vi "GPIO_RegChangeID.vi"(9 "GPIO Register New":T1, 11 "GPIO Register Old":T1) -> (1 "GPIO Reg Value":u32 format="%.0x", 3 "Command String":string)   [LabVIEW 2010]
doc: "This VI determines the GPIO data or direction bit that was change and creates the correct command string.\n\nInputs:\nGPIO Register Old - (cluster) previous value of GPIO register control\nGPIO Register New - (cluster) new value of GPIO register control\n\nOutputs:\nCommand String - (str) command for enqueue\n - for data bit change => \"GPIO Data Change:GPIODx\"\n - for direction bit change => \"GPIO Direction Change:GPIOCx\"\nGPIO Reg Value - (u32) GPIO regiter value"
uses:
  Controls/Register/TYP_Reg_GPIO.ctl
panel:
  out "GPIODx":u32
  out "GPIOCx":u32
  out "GPIODx Change?":bool caption="GPIODx Change? (or GPIOCx)"
  # "Out"
  # "IN"
  # "Out"
  # "IN"
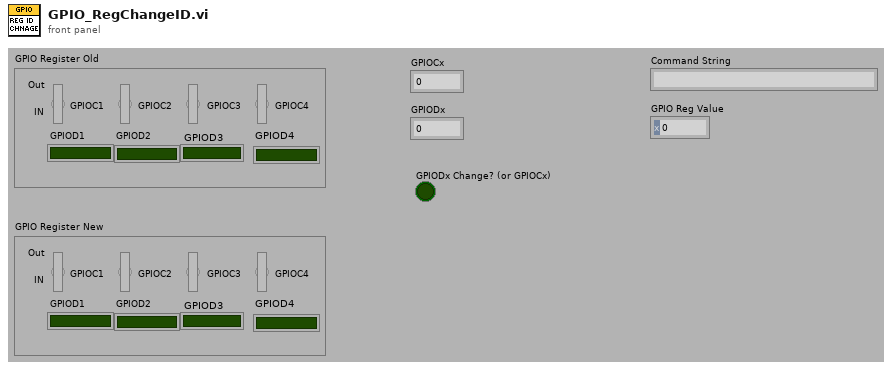
[diagram p1: front panel]
types:
  T1 = typedef "TYP_Reg_GPIO.ctl" = cluster{"GPIOC1":bool, "GPIOC2":bool, "GPIOC3":bool, "GPIOC4":bool, "GPIOD1":bool, "GPIOD2":bool, "GPIOD3":bool, "GPIOD4":bool}
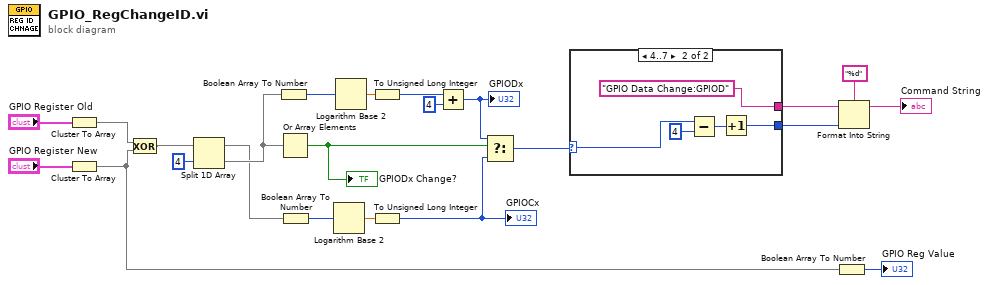
[diagram p0: block diagram]
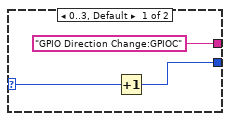
[diagram p2: hidden frame]
diagram:
  n1 = Cluster To Array(cluster="GPIO Register Old") -> (array=w14:bool[])
  n2 = Cluster To Array(cluster="GPIO Register New") -> (array=w2:bool[])
  n3 = Exclusive Or(1:w2, 2:w14) -> (0:w3:bool[])
  n4 = Split 1D Array(array=w3, index=4) -> (first subarray=w12:bool[], second subarray=w13:bool[])
  n5 = Boolean Array To Number(Boolean array=w13) -> (number=w20:u32)
  n6 = Or Array Elements(Boolean array=w13) -> (logical OR=w11:bool)
  "GPIODx Change?" <- w11
  n7 = Boolean Array To Number(Boolean array=w12) -> (number=w18:u32)
  n8 = Logarithm Base 2(1:w18) -> (0:w17:dbl)
  n9 = Logarithm Base 2(1:w20) -> (0:w19:dbl)
  n10 = To Unsigned Long Integer(number=w19) -> (unsigned 32bit integer=w16:u32)
  n11 = To Unsigned Long Integer(number=w17) -> (unsigned 32bit integer=w9:u32)
  "GPIOCx" <- w9
  n12 = Add(x=w16, y=u32 4) -> (x+y=w10:u32)
  "GPIODx" <- w10
  n13 = Select(t=w10, s=w11, f=w9) -> (s? t:f=w8:u32)
  n14 = case shown="4..7" w8 {
    selector: w8 -> [w26 w31]
    tunnel: [w25 w28] -> w7
    tunnel: ["GPIO Direction Change:GPIOC" "GPIO Data Change:GPIOD"] -> w6
    frame 0..3, Default {
      n15 = Increment(x=w26) -> (x+1=w25:u32)
    }
    frame 4..7 {
      n16 = Subtract(x=w31, y=u32 4) -> (x-y=w29:u32)
      n17 = Increment(x=w29) -> (x+1=w28:u32)
    }
  }
  n18 = Boolean Array To Number(Boolean array=w2) -> (number=→"GPIO Reg Value":u32)
  n19 = Format Into String(format string="%d", initial string=w6, w7) -> (resulting string=→"Command String":string)  [unwired: 1 in, 1 out]
